vi "19572_rs232_settings.vi"(8 "error in (no error)":errorcluster, 10 "input cluster":T1, 11 "reference in":refnum<visa-resource-name>) -> (0 "error out":errorcluster, 3 "reference out":refnum<visa-resource-name>)   [LabVIEW 2015]
uses:
  Type Definitions/get_visa_resources_data.ctl
  <vilib>/Instr/_visa.llb/VISA Configure Serial Port (Instr).vi
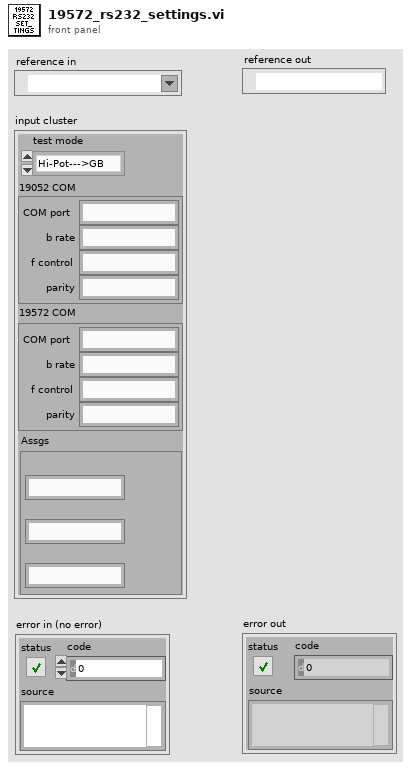
[diagram p1: front panel]
types:
  T1 = typedef "get_visa_resources_data.ctl" = cluster{"19052 COM":cluster{"COM port":string, "b rate":string, "f control":string, "parity":string}, "19572 COM":cluster{"COM port":string, "b rate":string, "f control":string, "parity":string}, "Assgs":cluster{"VISA1 Inst ID":string, "VISA2 Inst ID":string, "I/F type":string}, "test mode":enum16{"Hi-Pot--->GB", "GB--->Hi-Pot", "Hi-Pot only", "GB only"}}
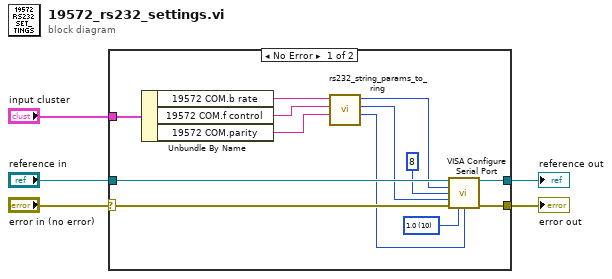
[diagram p0: block diagram]
diagram:
  n1 = case shown="No Error" "error in (no error)" {
    selector: "error in (no error)" -> [w18 w20]
    tunnel: "reference in" -> [w17 w19]
    tunnel: [w6 w19] -> w4
    tunnel: "input cluster" -> [w16 _]
    tunnel: [w7 w20] -> w2
    frame No Error {
      w8 = u16 10 items=["1.0"=10, "1.5"=15, "2.0"=20] ("stop bits (10: 1 bit)")
      n2 = Unbundle By Name(w16) -> ("19572 COM.b rate"=w15:string, "19572 COM.f control"=w14:string, "19572 COM.parity"=w13:string)
      n3 = call "rs232_string_params_to_ring.vi"("flow control string"=w13, "parity string"=w14, "baud rate string"=w15) -> ("Flow control"=w12:u16, "Parity"=w10:enum16{"None", "Odd", "Even", "Mark", "Space"}, "Baud rate"=w11:u32)  [unwired: 6 in]
      n4 = call-poly "VISA Configure Serial Port"("VISA resource name"=w17, "baud rate (9600)"=w11, "data bits (8)"=u16 8, "parity (0:none)"=w10, "error in (no error)"=w18, "stop bits (10: 1 bit)"=w8, "flow control (0:none)"=w12) -> ("VISA resource name out"=w6:refnum<visa-resource-name>, "error out"=w7:errorcluster)  [unwired: 7 in]
    }
    frame Error {
    }
  }
  "reference out" <- w4
  "error out" <- w2
